vi "VI-Add Event Data in Events.vi"(0 "XCtl Path in":path=path "C:/Users/Ken/Desktop/New XControl/New XControl.xctl", 7 "Event Data typedef":path=path "C:/Users/Ken/Desktop/New XControl/New Event Data.ctl", 11 "error in (no error)":errorcluster) -> (4 "XCtl Path out":path, 8 "Events typedef":path, 15 "error out":errorcluster)   [LabVIEW 2015]
uses:
  <vilib>/Utility/traverseref.llb/TRef TravTarget.ctl
  <vilib>/Utility/miscctls.llb/LVPositionTypeDef.ctl
  <vilib>/Utility/traverseref.llb/VI Scripting - Traverse.lvlib
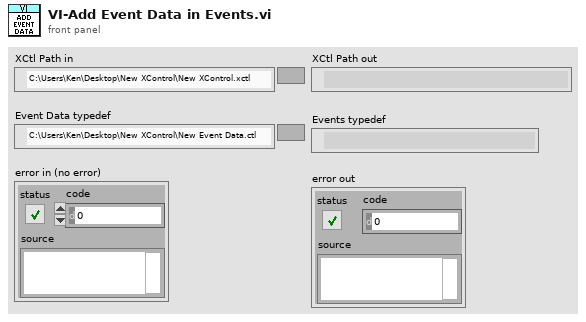
[diagram p1: front panel]
types:
  T1 = typedef "LVPositionTypeDef.ctl" = cluster{"Left":i32, "Top":i32}
  T2 = typedef "TRef TravTarget.ctl" = enum16{"FP", "BD", "Other"}
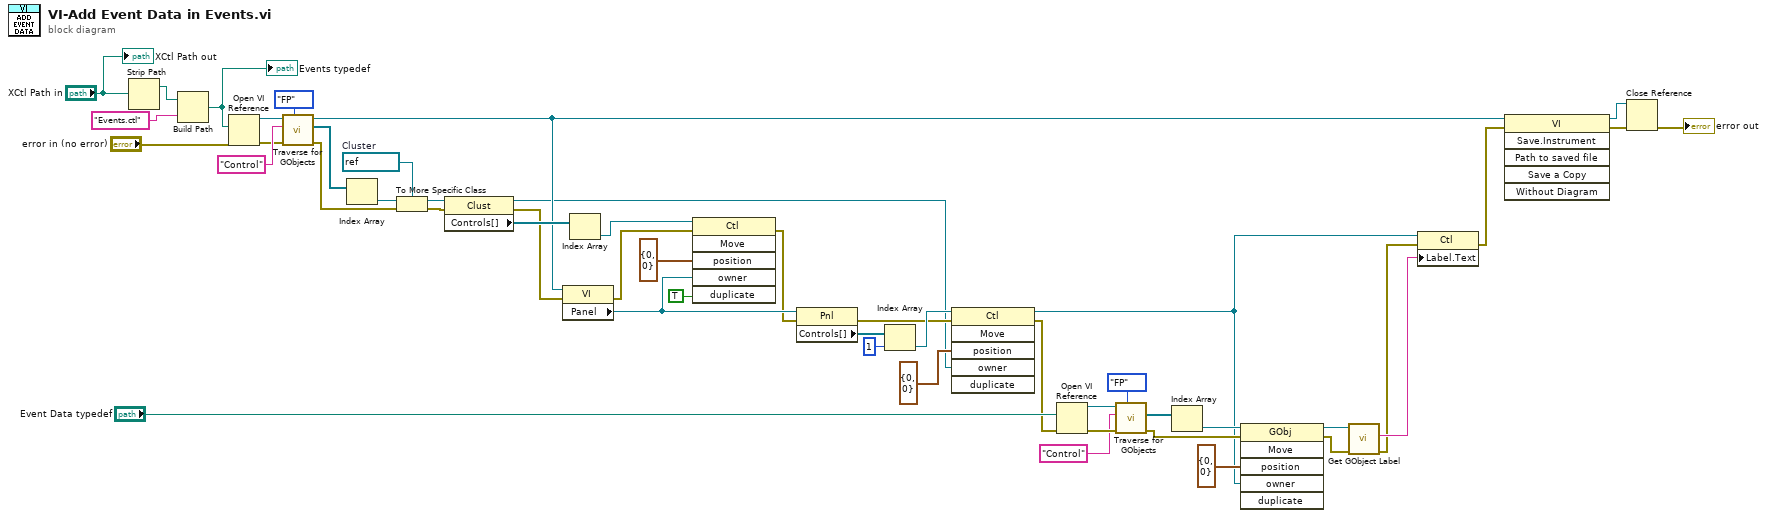
[diagram p0: block diagram]
diagram:
  w40 = refnum<vi> refnum  # Cluster
  n1 = Strip Path(path="XCtl Path in") -> (stripped path=w33:path)  [unwired: 1 out]
  n2 = Build Path(base path=w33, name or relative path="Events.ctl") -> (appended path=w31:path)
  "Events typedef" <- w31
  n3 = Open VI Reference(vi path=w31, error in (no error)="error in (no error)") -> (vi reference=w44:refnum<vi>, error out=w36:errorcluster)  [unwired: 4 in]
  n4 = call <vilib>:"Traverse for GObjects.vi"("Traverse Target"=TRef_TravTarget."FP", "error in (no error)"=w36, "Class Name"="Control", "VI Refnum"=w44) -> ("error out"=w37:errorcluster, "References"=w41:refnum<vi>[], "dup VI Refnum"=w13:refnum<vi>)  [unwired: 4 in, 1 out]
  n5 = Index Array(array=w41) -> (element=w30:refnum<vi>)  [unwired: 1 in]
  n6 = To More Specific Class(target class=w40, reference=w30, error in=w37) -> (specific class reference=w38:refnum<vi>, error out=w39:errorcluster)
  n7 = property class="Clust"(reference=w38, error in=w39) -> (reference out=w3:refnum<vi>, error out=w7:errorcluster, "Controls[]"=w45:refnum<vi>[])
  n8 = property class="VI"(reference=w13, error in=w7) -> (error out=w6:errorcluster, "Panel"=w12:refnum<vi>)  [unwired: 1 out]
  n9 = Index Array(array=w45) -> (element=w29:refnum<vi>)  [unwired: 1 in]
  n10 = invoke class="Ctl" method="Move"(reference=w29, error in=w6, "position"=T1 {"Left"=0, "Top"=0}, "owner"=w12, "duplicate"=TRUE ("Duplicate? (F)")) -> (error out=w5:errorcluster)  [unwired: 1 in, 5 out]
  n11 = property class="Pnl"(reference=w12, error in=w5) -> (error out=w4:errorcluster, "Controls[]"=w11:refnum<vi>[])  [unwired: 1 out]
  n12 = Index Array(array=w11, index=1) -> (element=w9:refnum<vi>)
  n13 = invoke class="Ctl" method="Move"(reference=w9, error in=w4, "position"=T1 {"Left"=0, "Top"=0}, "owner"=w3) -> (reference out=w1:refnum<vi>, error out=w2:errorcluster)  [unwired: 2 in, 4 out]
  n14 = Open VI Reference(vi path="Event Data typedef", error in (no error)=w2) -> (vi reference=w25:refnum<vi>, error out=w24:errorcluster)  [unwired: 4 in]
  n15 = call <vilib>:"Traverse for GObjects.vi"("Traverse Target"=TRef_TravTarget."FP", "error in (no error)"=w24, "Class Name"="Control", "VI Refnum"=w25) -> ("error out"=w20:errorcluster, "References"=w22:refnum<vi>[])  [unwired: 4 in, 2 out]
  n16 = Index Array(array=w22) -> (element=w19:refnum<vi>)  [unwired: 1 in]
  n17 = invoke class="GObj" method="Move"(reference=w19, error in=w20, "position"=T1 {"Left"=0, "Top"=0}, "owner"=w1) -> (reference out=w16:refnum<vi>, error out=w15:errorcluster)  [unwired: 2 in, 4 out]
  n18 = call <vilib>:"Get GObject Label.vi"("error in (no error)"=w15, "GObject"=w16) -> ("error out"=w14:errorcluster, "Object Label"=w18:string)  [unwired: 5 in, 3 out]
  n19 = property class="Ctl"(reference=w1, error in=w14, "Label.Text"=w18) -> (error out=w17:errorcluster)  [unwired: 1 out]
  n20 = invoke class="VI" method="Save.Instrument"(reference=w13, error in=w17) -> (reference out=w47:refnum<vi>, error out=w46:errorcluster)  [unwired: 4 in, 4 out]
  n21 = Close Reference(reference=w47, error in (no error)=w46) -> (error out=→"error out":errorcluster)
  "XCtl Path out" <- "XCtl Path in"
